vi "onHttpPatch (Buffer).vi"(8 "error in":errorcluster, 10 "httpRequest":refnum<class "httpRequest.lvclass">, 11 "REST Client in":refnum<class "REST Client.lvclass">) -> (0 "error out":errorcluster, 2 "httpResponse":refnum<class "httpResponse.lvclass">, 3 "REST Client out":refnum<class "REST Client.lvclass">)   [LabVIEW 2020, in "REST Client.lvlib" / "REST Client.lvclass"]
uses:
  REST Client.lvclass
  REST Client.lvclass/REST Client.ctl
  http-client-pkg/httpClient/httpClient.lvclass
  http-client-pkg/httpRequest/httpRequest.lvclass
  http-client-pkg/httpResponse/httpResponse.lvclass
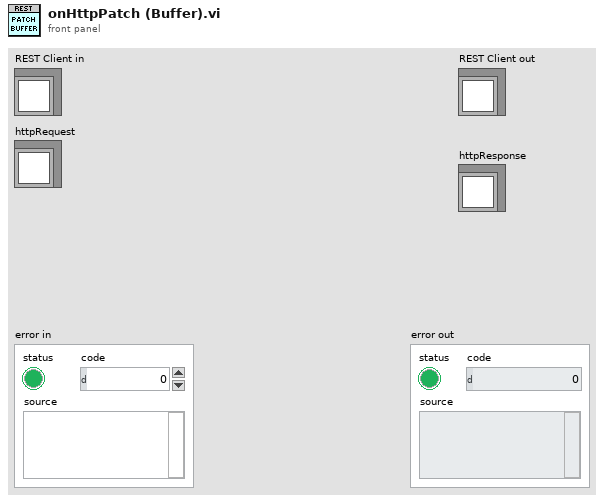
[diagram p1: front panel]
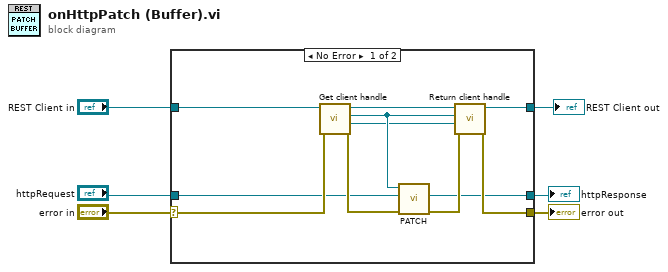
[diagram p0: block diagram]
diagram:
  n1 = case shown="No Error" "error in" {
    selector: "error in" -> [w12 w19]
    tunnel: [w10 w19] -> w3
    tunnel: [w11 w18] -> w4
    tunnel: "REST Client in" -> [w7 w18]
    tunnel: "httpRequest" -> [w8 _]
    tunnel: [w9 _] -> w5
    frame No Error {
      n2 = call "Get client handle.vi"("error in (no error)"=w12, "REST Client in"=w7) -> ("error out"=w14:errorcluster, "Headers dup"=w15:refnum<class "httpHeaders.lvclass">, "http-client"=w16:refnum<class "httpClient.lvclass">, "REST Client out"=w17:refnum<class "REST Client.lvclass">)  [unwired: 6 in]
      n3 = call "PATCH.vi"("error in"=w14, "httpRequest"=w8, "http-client in"=w16) -> ("error out"=w13:errorcluster, "httpResponse"=w9:refnum<class "httpResponse.lvclass">)  [unwired: 6 in, 1 out]
      n4 = call "Return client handle.vi"("error in (no error)"=w13, "Headers"=w15, "http-client"=w16, "REST Client in"=w17) -> ("error out"=w10:errorcluster, "REST Client out"=w11:refnum<class "REST Client.lvclass">)  [unwired: 6 in]
    }
    frame Error {
    }
  }
  "error out" <- w3
  "REST Client out" <- w4
  "httpResponse" <- w5
